vi "Destroy.vi"(0 "reference":refnum<class "GeneralPathEdge.lvclass">, 5 "error in (no error)":errorcluster) -> (15 "# of objects":i32, 19 "error out":errorcluster)   [LabVIEW 2012, in "GeneralPathEdge.lvclass"]
doc: "Destroys a GeneralPathEdge object created with a GeneralPathEdge constructor VI.\n\n[GOOP 2.1]"
uses:
  <resource>/Framework/Providers/Open_GDS/UML/GeneralPathEdge_class/GeneralPathEdge.lvclass
  <resource>/Framework/Providers/Open_GDS/UML/AbstractEdge_class/AbstractEdge.lvclass
panel:
  out "reference out":refnum<class "GeneralPathEdge.lvclass">
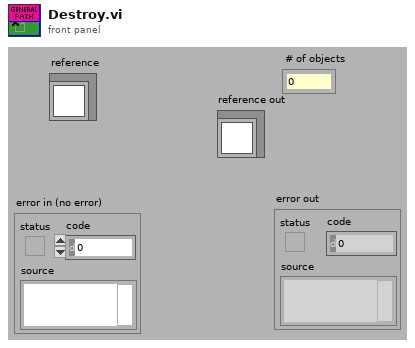
[diagram p1: front panel]
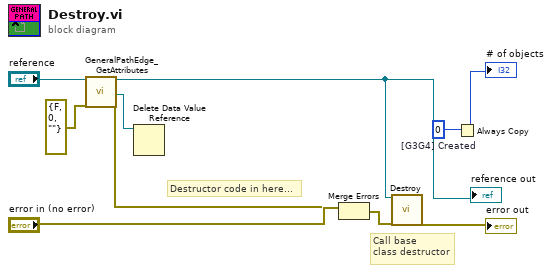
[diagram p0: block diagram]
diagram:
  w1 = 0  # [G3G4] Created
  # "Call base\nclass destructor"
  # "Destructor code in here..."
  n1 = call <resource>:"GeneralPathEdge_GetAttributes.vi"("reference in"="reference", "error in (no error)"=errorcluster {"status"=FALSE, "code"=0, "source"=""}) -> ("reference out"=w5:refnum<class "GeneralPathEdge.lvclass">, "DataRef"=w3:refnum<data-value>, "error out"=w6:errorcluster)  [unwired: 1 in, 14 out]
  "reference out" <- w5
  n2 = Delete Data Value Reference(data value reference=w3) -> ()  [unwired: 1 in, 2 out]
  n3 = Merge Errors("error in (no error)", w6) -> (w4:errorcluster)
  n4 = call-parent "Destroy.vi"("reference"=w5, "error in (no error)"=w4) -> ("error out"=→"error out":errorcluster)  [unwired: 16 in, 1 out]
  n5 = Always Copy(1:w1) -> (0:→"# of objects":i32)
